vi "Flock_Shared_Central Process Template.vi"() -> ()   [LabVIEW 2014]
uses:
  CentralProcessMessaging/Flock_Shared_CentralProcessMessaging.lvlib
  Flock_Shared_Messaging.lvlib
  ProcessList.ctl
  LocalProcessMessaging/Flock_Shared_LocalProcessMessaging.lvlib
  FA_AgentConfig API/source/VI Source/FA_AgentConfig.lvlib
  Error Handling/Flock_ErrorHandling.lvlib
panel:
  in  "Stop Button":bool
  in  "Dev":bool
  out "Status":string
  out "Idle Status":string
  # "Stop Button implementation is just for the template."
  # "Set as True if running Central Process in development environment"
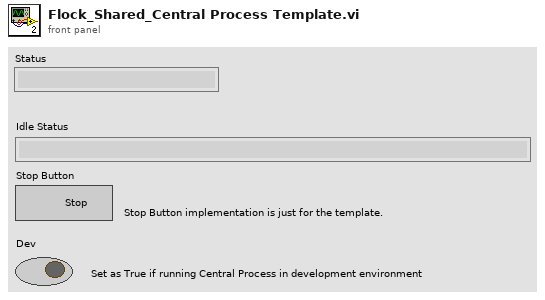
[diagram p1: front panel]
types:
  T1 = typedef "Flock_Shared_Messaging.lvlib/ProcessList.ctl" = string
  T2 = typedef "FA_AgentConfig.lvlib/FA_AgentConfig_Refnum.ctl" = cluster{"INI  Refnum":T3}
  T3 = typedef "NI_LVConfig.lvlib/Config Data RefNum.ctl" = refnum<k1>
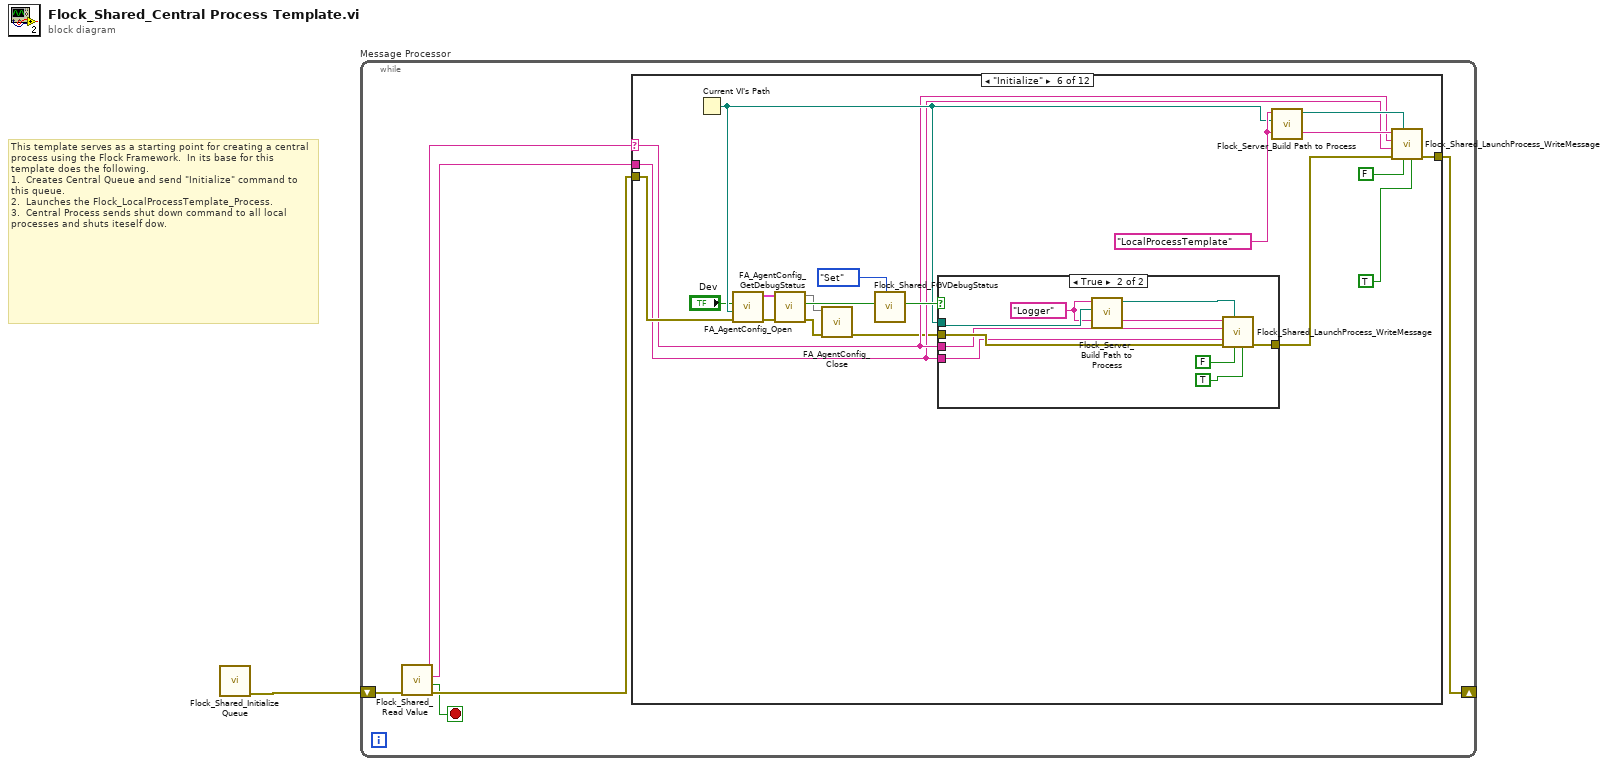
[diagram p0: block diagram]
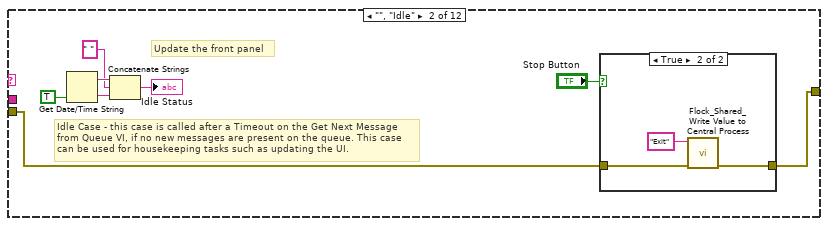
[diagram p3: hidden frame]
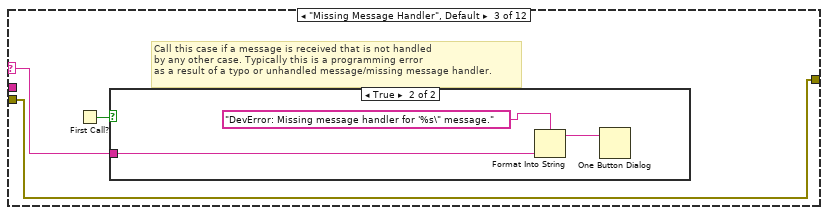
[diagram p5: hidden frame]
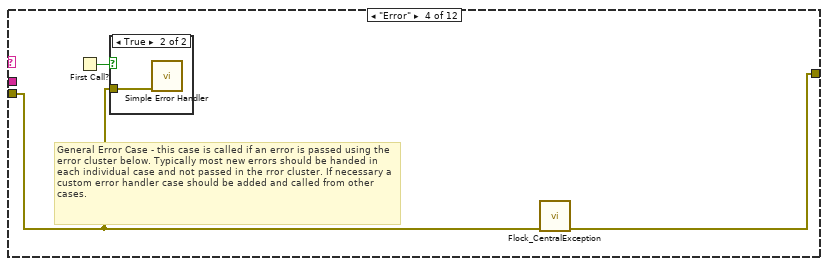
[diagram p7: hidden frame]
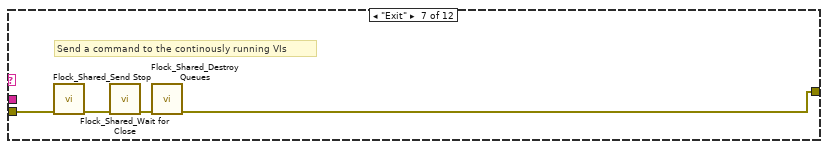
[diagram p11: hidden frame]
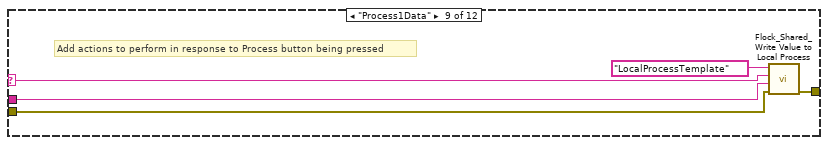
[diagram p13: hidden frame]
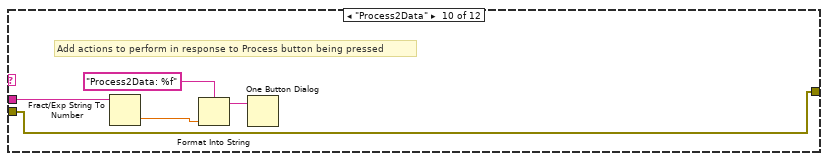
[diagram p14: hidden frame]
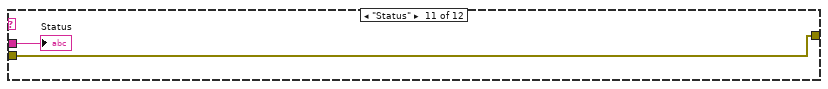
[diagram p15: hidden frame]
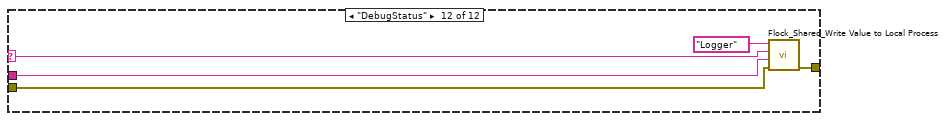
[diagram p16: hidden frame]
diagram:
  # "This template serves as a starting point for creating a central process using the Flock Framework.  In its base for this template does the following.\n1.  Creates Central Queue and send \"Initialize\" command to this queue.\n2.  Launches the Flock_LocalProcessTemplate_Process.\n3.  Central Process sends shut down command to all local processes and shuts iteself dow."
  n1 = call "Flock_Shared_Initialize Queue.vi"() -> ("error out"=w1:errorcluster)  [unwired: 11 in]
  n2 = while "Message Processor" {
    shift-left: w1 -> [w6]
    shift-right: [w7] -> _
    stop <- w4 stop-if-true
    n3 = call "Flock_Shared_Read Value.vi"("error in (no error)"=w6) -> ("error out"=w5:errorcluster, "Exit Process"=w4:bool, "Message Value"=w2:string, "Message Name"=w3:string)  [unwired: 7 in]
    n4 = case shown="\"Initialize\"" w3 {
      selector: w3 -> [_ _ w22 _ _ w36 _ _ w68 _ _ w82]
      tunnel: w5 -> [w8 w10 w23 w28 w31 w44 w63 w65 w70 w75 w76 w79]
      tunnel: [w8 w9 w23 w27 w31 w32 w64 w65 w67 w75 w76 w78] -> w7
      tunnel: w2 -> [_ _ _ _ _ w35 _ _ w69 w71 w77 w80]
      frame "---------- Framework Operations ----------" {
        # "Dummy case to add a seperator in the Case Structure menu"
      }
      frame "", "Idle" {
        # "Update the front panel"
        # "Idle Case - this case is called after a Timeout on the Get Next Message from Queue VI, if no new messages are present on the queue. This case can be used for housekeeping tasks such as updating the UI."
        n5 = Get Date/Time String(want seconds? (F)=TRUE) -> (date string=w16:string, time string=w15:string)  [unwired: 2 out]
        n6 = Concatenate Strings(w16, " " ("string"), w15) -> (→"Idle Status":string)
        n7 = case shown="True" "Stop Button" {
          tunnel: w10 -> [w17 w19]
          tunnel: [w17 w18] -> w9
          frame False {
          }
          frame True {
            n8 = call "Flock_Shared_Write Value to Central Process.vi"("error in (no error)"=w19, "Message Name"="Exit") -> ("error out"=w18:errorcluster)  [unwired: 9 in]
          }
        }
      }
      frame "Missing Message Handler", Default {
        # "Call this case if a message is received that is not handled \nby any other case. Typically this is a programming error\nas a result of a typo or unhandled message/missing message handler."
        n9 = First Call?() -> (First Call?: T/F=w21:bool)
        n10 = case shown="True" w21 {
          tunnel: w22 -> [_ w26]
          frame False {
          }
          frame True {
            n11 = Format Into String(format string="DevError: Missing message handler for '%s\" message." ("message"), w26) -> (resulting string=w24:string)  [unwired: 2 in, 1 out]
            n12 = One Button Dialog(message=w24) -> ()  [unwired: 2 out]
          }
        }
      }
      frame "Error" {
        # "General Error Case - this case is called if an error is passed using the error cluster below. Typically most new errors should be handed in each individual case and not passed in the rror cluster. If necessary a custom error handler case should be added and called from other cases."
        n13 = First Call?() -> (First Call?: T/F=w29:bool)
        n14 = case shown="True" w29 {
          tunnel: w28 -> [_ w30]
          frame False {
          }
          frame True {
            n15 = call <vilib>:"Simple Error Handler.vi"("error in (no error)"=w30) -> ()  [unwired: 1 in, 8 out]
          }
        }
        n16 = call "Flock_CentralException.vi"("Error In"=w28) -> ("Error Out"=w27:errorcluster)  [unwired: 10 in]
      }
      frame "---------- Generic Operations ----------" {
        # "Dummy case to add a seperator in the Case Structure menu"
      }
      frame "Initialize" {
        w47 = T1 "LocalProcessTemplate" ("Process")
        n17 = Current VI's Path() -> (path=w38:path)
        n18 = call "FA_AgentConfig_Open.vi"("Error In"=w44, "Current VI Path"=w38, "Dev"="Dev") -> ("Error Out"=w43:errorcluster, "INI File Path"=w39:T2)  [unwired: 7 in]
        n19 = call "FA_AgentConfig_GetDebugStatus.vi"("Error In"=w43, 11:w39) -> ("Error Out"=w42:errorcluster, "DebugStatus"=w46:bool, 3:w40)  [unwired: 7 in]
        n20 = call "FA_AgentConfig_Close.vi"("Error In"=w42, "FA_AgentConfig_Refnum 2"=w40) -> ("Error Out"=w34:errorcluster)  [unwired: 9 in]
        n21 = call "Flock_Shared_FGVDebugStatus.vi"("State"=enum16{"Get", "Set"}."Set", "DebugBoolean"=w46) -> ("Debug Boolean"=w41:bool)  [unwired: 9 in]
        n22 = case shown="True" w41 {
          tunnel: w38 -> [_ w60]
          tunnel: w34 -> [w51 w57]
          tunnel: [w51 w56] -> w33
          tunnel: w36 -> [_ w53]
          tunnel: w35 -> [_ w52]
          frame False {
          }
          frame True {
            w58 = T1 "Logger" ("Process")
            n23 = call "Flock_Server_Build Path to Process.vi"("path"=w60, "Process"=w58) -> ("Local Process Path"=w59:path)  [unwired: 9 in]
            n24 = call "Flock_Shared_LaunchProcess_WriteMessage.vi"("Show Front Panel?"=TRUE, "Reentrant?"=FALSE, "VI Path"=w59, "error in (no error)"=w57, "Initial Message Value"=w52, "Initial Message Name"=w53, "Process List"=w58) -> ("error out"=w56:errorcluster)  [unwired: 4 in]
          }
        }
        n25 = call "Flock_Server_Build Path to Process.vi"("path"=w38, "Process"=w47) -> ("Local Process Path"=w50:path)  [unwired: 9 in]
        n26 = call "Flock_Shared_LaunchProcess_WriteMessage.vi"("Show Front Panel?"=TRUE, "Reentrant?"=FALSE, "VI Path"=w50, "error in (no error)"=w33, "Initial Message Value"=w35, "Initial Message Name"=w36, "Process List"=w47) -> ("error out"=w32:errorcluster)  [unwired: 4 in]
      }
      frame "Exit" {
        # "Send a command to the continously running VIs"
        n27 = call "Flock_Shared_Send Stop.vi"("error in (no error)"=w63) -> ("error out"=w62:errorcluster)  [unwired: 10 in]
        n28 = call "Flock_Shared_Wait for Close.vi"("error in (no error)"=w62) -> ("error out"=w61:errorcluster)  [unwired: 10 in]
        n29 = call "Flock_Shared_Destroy Queues.vi"("error in (no error)"=w61) -> ("error out"=w64:errorcluster)  [unwired: 10 in]
      }
      frame "---------- Application Operations ----------" {
        # "Dummy case to add a seperator in the Case Structure menu"
      }
      frame "Process1Data" {
        # "Add actions to perform in response to Process button being pressed"
        n30 = call "Flock_Shared_Write Value to Local Process.vi"("error in (no error)"=w70, "Message Value"=w69, "Message Name"=w68, "Process List"=T1 "LocalProcessTemplate" ("Process")) -> ("error out"=w67:errorcluster)  [unwired: 7 in]
      }
      frame "Process2Data" {
        # "Add actions to perform in response to Process button being pressed"
        n31 = Fract/Exp String To Number(string=w71) -> (number=w74:dbl)  [unwired: 4 out]
        n32 = Format Into String(format string="Process2Data: %f" ("message"), w74) -> (resulting string=w72:string)  [unwired: 2 in, 1 out]
        n33 = One Button Dialog(message=w72) -> ()  [unwired: 2 out]
      }
      frame "Status" {
        "Status" <- w77
      }
      frame "DebugStatus" {
        n34 = call "Flock_Shared_Write Value to Local Process.vi"("error in (no error)"=w79, "Message Value"=w80, "Message Name"=w82, "Process List"=T1 "Logger" ("Process")) -> ("error out"=w78:errorcluster)  [unwired: 7 in]
      }
    }
  }
